vi "CheckCA.vi"(0 "data":i16[][](array[numeric]), 1 "valid peak in":i32[](array[numeric]), 3 "Voltage Scale":u16, 5 "count in":i32, 9 "Dig Word Size":u16, 11 "fill array":i16[][](array[numeric]), 12 "Digitizer Settings":T1={"Digitizer delay (us) "=0.0, "rf points per line"=2048, "lines per plane"=128, "Samp Rate (Hz)"=100000000.0, "Additional dig delay (us)"=0.0, "Voltage Scale"=0.4, "Pre-Looks"=0, "Offset delay (us)"=0.0, "bits A/D"=8, "Avg Num"=1, "DigTimeOut"=5.0, "Rel Dig Delay"=0.0, "Dig Ch"=0, "LeCroyCluster"={"LeCroy Channels"=[TRUE, FALSE, FALSE, FALSE], "LC read pt offset"=0.0, "Sweep Avg"=FALSE}, "Main Digitizer"=enum."NI Digitizer", "Dig Config"=enum."Single channel", "Digitizer ID Cluster"={"Acqiris/Alazar/SP ID"=[], "NI Instr Handles"=[], "LeCroy VISA"="", "GaGe Handle"={"Handle"=0, "Sample size"=0, "Resolution"=0, "Offset"=0, "Channels"=0, "Boards"=0}, "ATS Ref"="ATS9350", "Acqiris Address"=["PCI::INSTR0"], "ADQRef"=refnum, "adq_cu_ptr"=refnum}, "Trigger Settings"={"Trig Source"=1, "Trig Coupling"=0, "Trig Slope"=0, "Level (mV)"=1500.0}, "Bulk Acq"=FALSE, "Bulk Start Indexes"=[], "Data Ref RF"=refnum, "NI ID/Channel"=[], "Total Dig CH"=1, "Xtra Ann Trig delay (us)"=10.0, "Fix Z Delay?"=FALSE, "One Way Transmission?"=FALSE, "Data Ref Log"=refnum} {"Trigger Settings"."Trig Slope" items=["Positive", "Negative"]; "Trigger Settings"."Level (mV)" format="%.2f"; "Trigger Settings"."Trig Coupling" items=["DC 1 MOhm", "AC 1 MOhm", "DC 50 Ohm", "AC 50 Ohm"]; "Trigger Settings"."Trig Source" items=["Chan 1", "External"]; "Rel Dig Delay" format="%.2f"; "DigTimeOut" format="%.2f"; "Avg Num" min=1; "Offset delay (us)" format="%.2f"; "Additional dig delay (us)" format="%.2f"; "Digitizer delay (us)" format="%.2f"}, 13 "CA Threshold":i16=62) -> (4 "valid peak out":i32[](array[numeric]), 6 "count out":i32, 10 "All peaks":i32, 14 "valild peak line":i32, 15 "fill out":i16[][](array[numeric]))   [LabVIEW 2022 SP3]
uses:
  Digitizers/-DigitizerRoutines/DigitizerSettings.ctl
  Digitizers/-DigitizerRoutines/Digitizer.ctl
  Digitizers/-DigitizerRoutines/DigConfig.ctl
  Digitizers/-DigitizerRoutines/DigitizerID.ctl
  C:/Windows/System32/ADQAPI_dotNet_helper.dll
  <vilib>/Analysis/2dsp.llb/1D Convolution (DBL).vi
  <vilib>/Analysis/baseanly.llb/Mean (DBL).vi
  <vilib>/Analysis/baseanly.llb/Quick Scale 1D.vi
  Motion Controllers/-MotionRoutines/MotionGlobals.vi
  Pulsers/PulserGlobals.vi
  <vilib>/Analysis/2dsp.llb/1D Cross Correlation (DBL).vi
  <vilib>/Analysis/NI_AALBase.lvlib
  <vilib>/Analysis/NI_AALPro.lvlib
panel:
  out "RF mean":dbl format="%0.2f"
  out "CA Line":cluster{"element":dbl, dbl, "data":i16[]}(graph)
  in  "width":i32=15 min=3
  out "M-mode":i16[][](graph)
  in  "falsify hit?":bool
  in  "View Acq?":bool
  in  "+/- search window":i16=125
  # "use this to generate dummy data and get through acquisition"
  # "Current count of hits"
  # "Current peak"
  # "Line of valid\npeak"
  # "Theshold scales with voltage range"
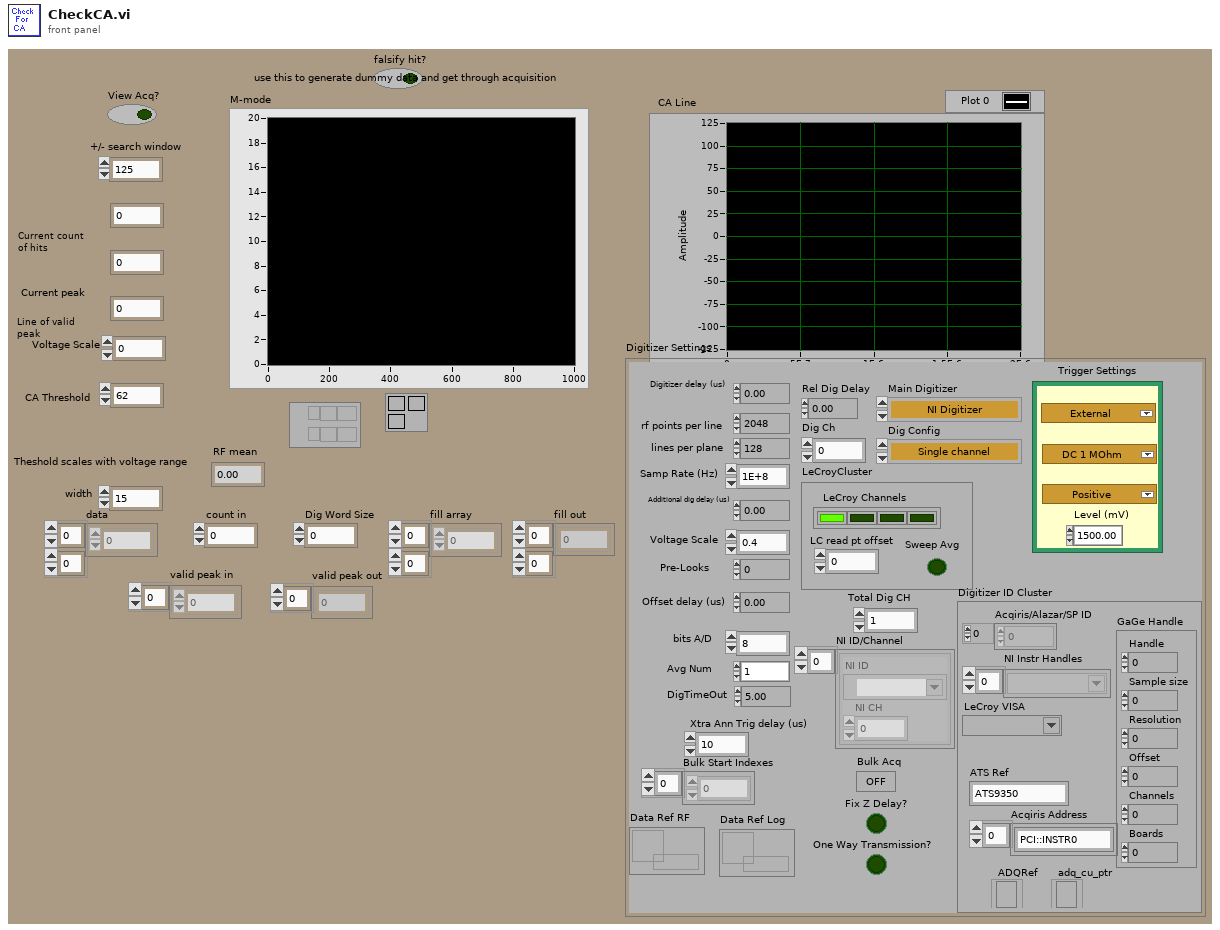
[diagram p1: front panel]
types:
  T1 = typedef "DigitizerSettings.ctl" = cluster{"Digitizer delay (us) ":dbl, "rf points per line":i32, "lines per plane":i32, "Samp Rate (Hz)":dbl, "Additional dig delay (us)":dbl, "Voltage Scale":dbl, "Pre-Looks":i32, "Offset delay (us)":dbl, "bits A/D":i8, "Avg Num":i32, "DigTimeOut":sgl, "Rel Dig Delay":sgl, "Dig Ch":i32, "LeCroyCluster":cluster{"LeCroy Channels":bool[], "LC read pt offset":dbl, "Sweep Avg":bool}, "Main Digitizer":T2, "Dig Config":T3, "Digitizer ID Cluster":T4, "Trigger Settings":cluster{"Trig Source":u16, "Trig Coupling":u16, "Trig Slope":u16, "Level (mV)":dbl}, "Bulk Acq":bool, "Bulk Start Indexes":i32[], "Data Ref RF":refnum<data-value>, "NI ID/Channel":cluster{"NI ID":refnum<k15>, "NI CH":i32}[], "Total Dig CH":i32, "Xtra Ann Trig delay (us)":dbl, "Fix Z Delay?":bool, "One Way Transmission?":bool, "Data Ref Log":refnum<data-value>}
  T2 = typedef "Digitizer.ctl" = enum16{"Acqiris Digitizer", "NI Digitizer", "LeCroy", "GaGe", "AlazarTech", "No Digitizer", "Teledyne"}
  T3 = typedef "DigConfig.ctl" = enum16{"Single channel", "2 Chans w/ 2 Acqiris", "2 Chans w/ 1 Acqiris", "5-CH Pulser New", "5-CH pulser w/ ann array", "5-pass style ann array", "Empty"}
  T4 = typedef "DigitizerID.ctl" = cluster{"Acqiris/Alazar/SP ID":u32[], "NI Instr Handles":refnum<k15>[], "LeCroy VISA":refnum<visa-resource-name>, "GaGe Handle":cluster{"Handle":u32, "Sample size":u32, "Resolution":i32, "Offset":i32, "Channels":u32, "Boards":u32}, "ATS Ref":string, "Acqiris Address":string[], "ADQRef":refnum<k24>, "adq_cu_ptr":refnum<k24>}
  T5 = cluster{"Therapy frequency (MHz)":dbl, "Therapy amplitude (mV)":dbl, "time therapy on (s)":dbl, "Therapy Delay (ms) ":dbl, "Time (s)":dbl}
  T6 = cluster{"F1 (MHz)":sgl, "F2 (MHz)":sgl, "Tukey taper":sgl, "duration":sgl}
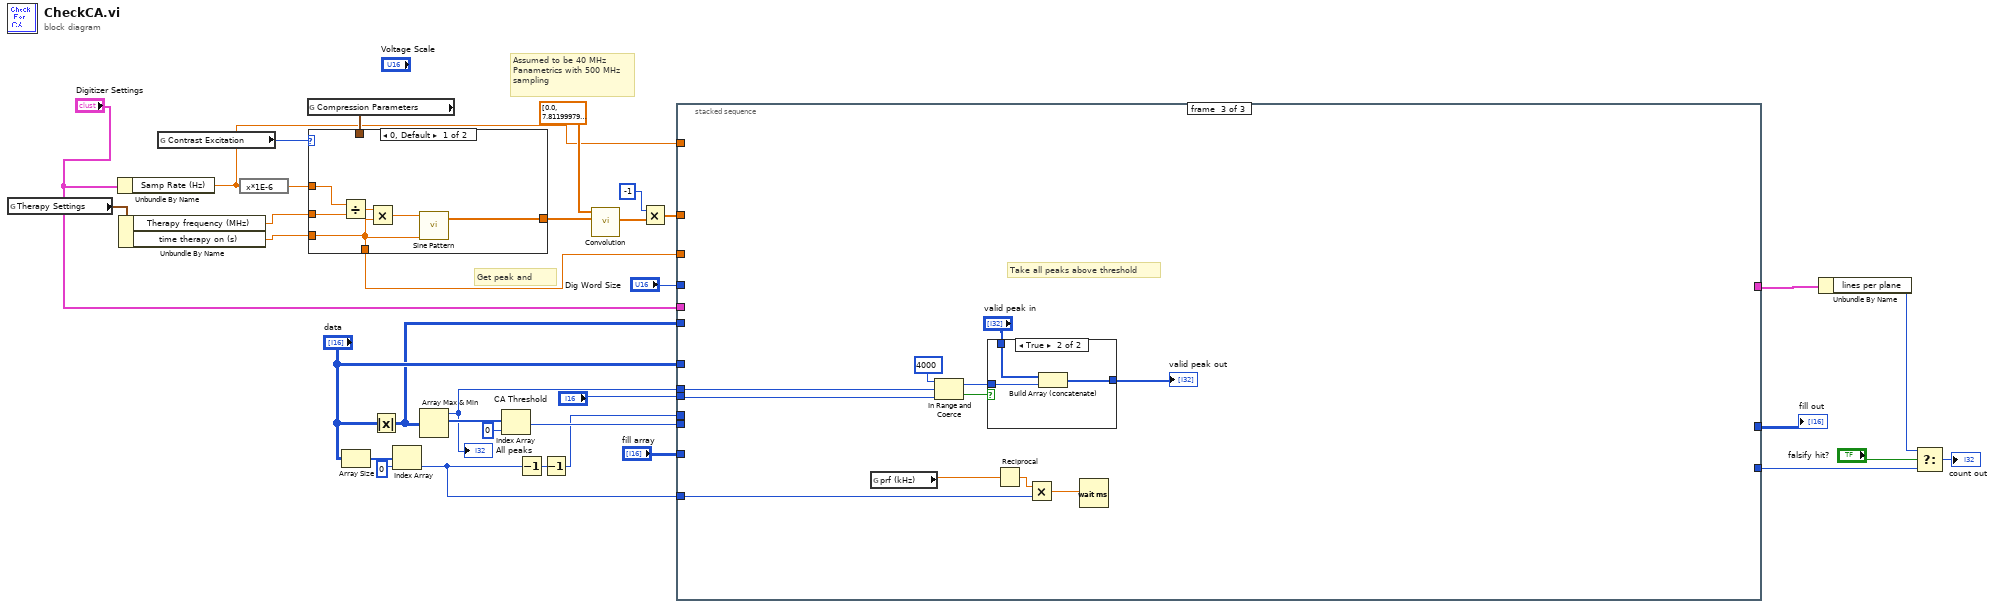
[diagram p0: block diagram]
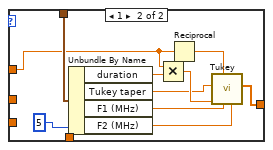
[diagram p2: hidden frame]
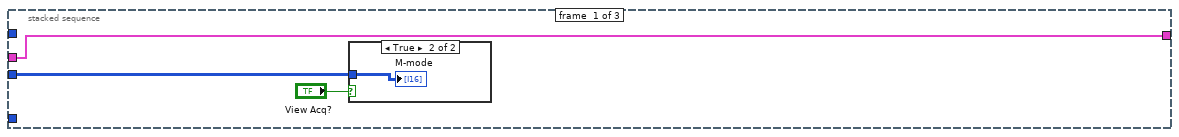
[diagram p3: hidden frame]
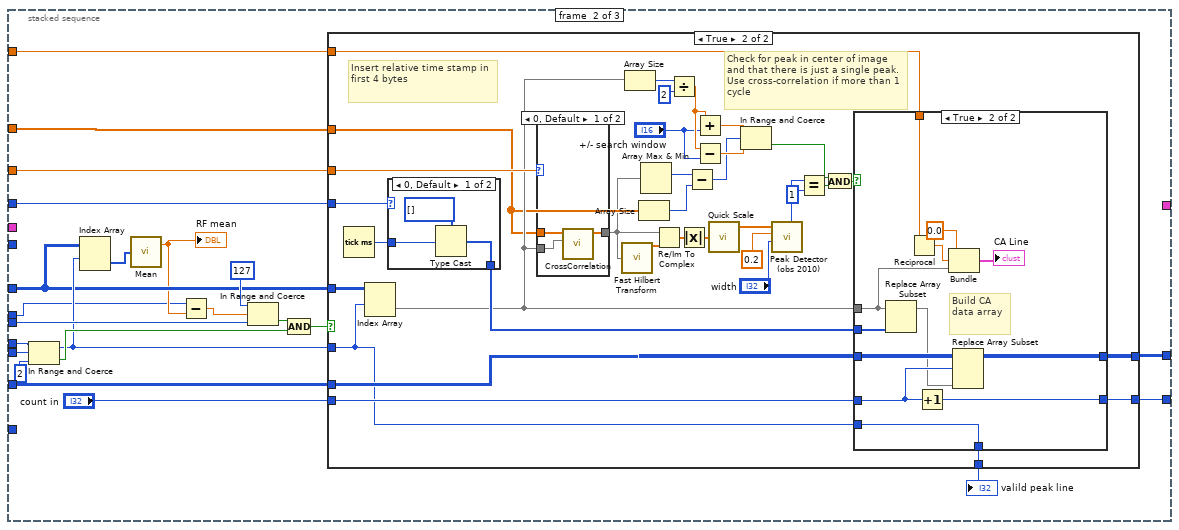
[diagram p5: hidden frame]
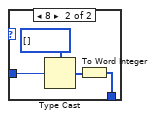
[diagram p9: hidden frame]
diagram:
  # "Get peak and"
  # "Assumed to be 40 MHz Panametrics with 500 MHz  sampling"
  n1 = global read "PulserGlobals.vi" "Therapy Settings"() -> (w3:T5)
  n2 = Unbundle By Name("Digitizer Settings") -> ("Samp Rate (Hz)"=w8:dbl)
  n3 = Unbundle By Name(w3) -> ("Therapy frequency (MHz)"=w2:dbl, "time therapy on (s)"=w1:dbl)
  n4 = global read "PulserGlobals.vi" "Contrast Excitation"() -> (w4:u16)
  n5 = expression code="x*1E-6"(w8) -> (w10:dbl)
  n6 = global read "MotionGlobals.vi" "Compression Parameters"() -> (w13:T6)
  n7 = case shown="0, Default" w4 {
    tunnel: w2 -> [w38 _]
    tunnel: w1 -> [w35 _]
    tunnel: w10 -> [w37 w43]
    tunnel: [w36 w42] -> w9
    tunnel: w13 -> [_ w44]
    tunnel: [w35 5] -> w11
    frame 0, Default {
      n8 = Divide(x=w37, y=w38) -> (x/y=w40:dbl)
      n9 = Multiply(x=w40, y=w35) -> (x*y=w39:dbl)
      n10 = call <vilib>:"Sine Pattern.vi"("cycles"=w35, "samples"=w39) -> ("Sinusoidal Pattern"=w36:dbl[])  [unwired: 2 in, 1 out]
    }
    frame 1 {
      n11 = Unbundle By Name(w44) -> ("duration"=w50:sgl, "Tukey taper"=w45:sgl, "F1 (MHz)"=w49:sgl, "F2 (MHz)"=w48:sgl)
      n12 = Multiply(x=w43, y=w50) -> (x*y=w46:dbl)
      n13 = Reciprocal(x=w43) -> (1/x=w47:dbl)
      n14 = call "Tukey.vi"("f2 (MHz)"=w48, "f1 (MHz)"=w49, "Samp Rate (mics)"=w47, "Pts"=w46, "Tukey"=w45) -> ("Tukey Chirp"=w42:dbl[])  [unwired: 2 in, 4 out]
    }
  }
  n15 = Array Size(array="data") -> (size(s)=w26:i32[])
  n16 = Absolute Value(x="data") -> (abs(x)=w17:i16[][])
  n17 = Index Array(array=w26, index=0) -> (element=w16:i32)
  n18 = Array Max & Min(array=w17) -> (max value=w21:i16, max index (indices)=w29:i32[])  [unwired: 2 out]
  "All peaks" <- w21
  n19 = Index Array(array=w29, index=0) -> (element=w19:i32)
  n20 = Decrement(x=w16) -> (x-1=w34:i32)
  n21 = Decrement(x=w34) -> (x-1=w18:i32)
  n22 = call-poly <vilib>:"Convolution.vi"("Y"=w9, "X"=sgl[] [0.0, 7.812, 7.812, 0.0, 0.0, -15.625, -31.25, -46.875, -31.25, 31.25, 132.812, 257.812, 328.125, 304.687, 179.687, -31.25, -257.812, -421.875, -484.375, -468.75, -406.25, -289.062, -93.75, 210.937, 562.5, 812.5, 851.562, 664.062, 250.0, -210.937, -578.125, -742.187, -703.125, -484.375, -218.75, 31.25, 281.25, 468.75, 515.625, 421.875, 210.937, -39.062, -218.75, -304.687, -296.875, -218.75, -101.562, 0.0, 109.375, 187.5, 218.75, 195.312, 132.812, 54.687, -7.812, -54.687, -70.312, -62.5, -31.25, 0.0, 39.062, 62.5, 85.937, 93.75, 78.125, 46.875, 23.437, -7.812, -15.625, -15.625, -23.437, -15.625, 7.812, 7.812, 15.625, 31.25, 15.625, 15.625, 7.812, 0.0, -7.812, -7.812, -7.812, 0.0, -7.812] ("decimated array")) -> ("X * Y"=w14:dbl[])  [unwired: 1 in, 8 out]
  n23 = Multiply(x=-1, y=w14) -> (x*y=w15:dbl[])
  n24 = stacked-sequence {
    tunnel: "Dig Word Size" -> [_ w75 _]
    tunnel: [_ w74 _] -> w31
    tunnel: "fill array" -> [_ w73 _]
    tunnel: "data" -> [_ w59 _]
    tunnel: w11 -> [_ w72 _]
    tunnel: w15 -> [_ w71 _]
    tunnel: [_ w70 _] -> w23
    tunnel: w21 -> [_ w56 w146]
    tunnel: "CA Threshold" -> [_ w68 w147]
    tunnel: w19 -> [_ w65 _]
    tunnel: w18 -> [_ w64 _]
    tunnel: w17 -> [w53 _ _]
    tunnel: w16 -> [_ _ w149]
    tunnel: w8 -> [_ w62 _]
    tunnel: "Digitizer Settings" -> [w51 _ _]
    tunnel: [w51 _ _] -> w7
    frame #0 {
      n25 = case shown="True" "View Acq?" {
        tunnel: w53 -> [_ w54]
        frame False {
        }
        frame True {
          "M-mode" <- w54
        }
      }
    }
    frame #1 {
      n26 = In Range and Coerce(upper limit=w64, x=w65, lower limit=2) -> (coerced(x)=w60:i32, In Range?=w66:bool)
      n27 = Index Array(array=w59, index (row)=w60) -> (element=w58:i16[])  [unwired: 1 in]
      n28 = call-poly <vilib>:"Mean.vi"("X"=w58) -> ("mean"=w57:dbl)  [unwired: 1 out]
      "RF mean" <- w57
      n29 = Subtract(x=w56, y=w57) -> (x-y=w55:dbl)
      n30 = In Range and Coerce(upper limit=127, x=w55, lower limit=w68) -> (In Range?=w67:bool)  [unwired: 1 out]
      n31 = Compound Arithmetic op=AND(w67, w66) -> (w77:bool)
      n32 = case shown="True" w77 {
        tunnel: w73 -> [w79 w113]
        tunnel: [w79 w112] -> w74
        tunnel: w59 -> [_ w114]
        tunnel: w60 -> [_ w80]
        tunnel: "count in" -> [w78 w107]
        tunnel: [w78 w111] -> w70
        tunnel: w75 -> [_ w108]
        tunnel: w71 -> [_ w90]
        tunnel: w72 -> [_ w102]
        tunnel: w62 -> [_ w82]
        tunnel: [_ w81] -> w61
        frame False {
        }
        frame True {
          # "Check for peak in center of image and that there is just a single peak. Use cross-correlation if more than 1 cycle"
          # "Insert relative time stamp in first 4 bytes"
          n33 = Tick Count (ms)() -> (millisecond timer value=w110:u32)
          n34 = Index Array(array=w114, index (row)=w80) -> (element=w91:i16[])  [unwired: 1 in]
          n35 = case shown="0, Default" w108 {
            tunnel: w110 -> [w135 w139]
            tunnel: [w134 w136] -> w109
            frame 0, Default {
              n36 = Type Cast(type=i16[] [], x=w135) -> (*(type *) &x=w134:i16[])
            }
            frame 8 {
              n37 = Type Cast(type=i8[] [], x=w139) -> (*(type *) &x=w137:i8[])
              n38 = To Word Integer(number=w137) -> (16bit integer=w136:i16[])
            }
          }
          n39 = case shown="0, Default" w102 {
            tunnel: w90 -> [w117 _]
            tunnel: w91 -> [w116 w118]
            tunnel: [w115 w118] -> w85
            frame 0, Default {
              n40 = call-poly <vilib>:"CrossCorrelation.vi"("Y"=w116, "X"=w117) -> ("Rxy"=w115:dbl[])  [unwired: 2 in, 7 out]
            }
            frame 1 {
            }
          }
          n41 = call <vilib>:"Fast Hilbert Transform.vi"("X"=w85) -> ("Hilbert{X}"=w98:dbl[])  [unwired: 1 out]
          n42 = Array Size(array=w91) -> (size(s)=w104:i32)
          n43 = Array Size(array=w90) -> (size(s)=w87:i32)
          n44 = Array Max & Min(array=w85) -> (max index (indices)=w89:i32)  [unwired: 3 out]
          n45 = Re/Im To Complex(1:w98, 2:w85) -> (0:w99:cdb[])
          n46 = Divide(x=w104, y=2) -> (x/y=w103:dbl)
          n47 = Absolute Value(x=w99) -> (abs(x)=w83:dbl[])
          n48 = Subtract(x=w89, y=w87) -> (x-y=w88:i32)
          n49 = Add(x=w103, y="+/- search window") -> (x+y=w100:dbl)
          n50 = Subtract(x=w103, y="+/- search window") -> (x-y=w105:dbl)
          n51 = call-poly <vilib>:"Quick Scale.vi"("X"=w83) -> ("Y[i]=X[i]/Max|X|"=w84:dbl[])  [unwired: 2 out]
          n52 = In Range and Coerce(upper limit=w100, x=w88, lower limit=w105) -> (In Range?=w94:bool)  [unwired: 1 out]
          n53 = call <vilib>:"Peak Detector (obs 2010).vi"("width"="width", "threshold"=0.2, "X"=w84) -> ("# found"=w97:i32)  [unwired: 4 in, 4 out]
          n54 = Equal?(x=w97, y=1) -> (x = y?=w95:bool)
          n55 = And(x=w94, y=w95) -> (x .and. y?=w93:bool)
          n56 = case shown="True" w93 {
            tunnel: w113 -> [w119 w132]
            tunnel: [w119 w131] -> w112
            tunnel: [w120 w130] -> w111
            tunnel: w109 -> [_ w129]
            tunnel: w107 -> [w120 w128]
            tunnel: w91 -> [_ w124]
            tunnel: w82 -> [_ w123]
            tunnel: [_ w121] -> w81
            tunnel: w80 -> [_ w121]
            frame False {
            }
            frame True {
              # "Build CA data array"
              n57 = Replace Array Subset(array=w124, new element=w129) -> (w127:i16[])  [unwired: 1 in]
              n58 = Reciprocal(x=w123) -> (1/x=w126:dbl)
              n59 = Increment(x=w128) -> (x+1=w130:i32)
              n60 = Bundle("element"=0.0, w126, "data"=w124) -> (→"CA Line":cluster{"element":dbl, dbl, "data":i16[]})  [unwired: 1 out]
              n61 = Replace Array Subset(array=w132, new element=w127, index (row)=w128) -> (w131:i16[][])  [unwired: 1 in]
            }
          }
        }
      }
      "valild peak line" <- w61
    }
    frame #2 {
      # "Take all peaks above threshold"
      n62 = global read "PulserGlobals.vi" "prf (kHz)"() -> (w140:dbl)
      n63 = In Range and Coerce(upper limit=i16 4000, x=w146, lower limit=w147) -> (coerced(x)=w143:i16, In Range?=w144:bool)
      n64 = case shown="True" w144 {
        tunnel: w143 -> [_ w154]
        tunnel: "valid peak in" -> [w151 w153]
        tunnel: [w151 w152] -> w141
        frame False {
        }
        frame True {
          n65 = Build Array (concatenate)(w153, w154) -> (w152:i32[])
        }
      }
      "valid peak out" <- w141
      n66 = Reciprocal(x=w140) -> (1/x=w150:dbl)
      n67 = Multiply(x=w150, y=w149) -> (x*y=w148:dbl)
      n68 = Wait (ms)(milliseconds to wait=w148) -> ()  [unwired: 1 out]
    }
  }
  "fill out" <- w31
  n69 = Unbundle By Name(w7) -> ("lines per plane"=w6:i32)
  n70 = Select(t=w6, s="falsify hit?", f=w23) -> (s? t:f=→"count out":i32)
